vi "Check States.vi"(8 "error in (no error)":refnum<class "MultiErrors.lvclass">, 11 "Sequence Validation in":refnum<class "Sequence Validation.lvclass">) -> (0 "error out":refnum<class "MultiErrors.lvclass">, 3 "Sequence Validation out":refnum<class "Sequence Validation.lvclass">)   [LabVIEW 2020, in "VolatusSeq.lvlib" / "Sequence Validation.lvclass"]
uses:
  Sequence Validation.lvclass
  Sequence Validation.lvclass/Sequence Validation.ctl
  VolatusErrorUtilities/MultiErrors/MultiErrors.lvclass
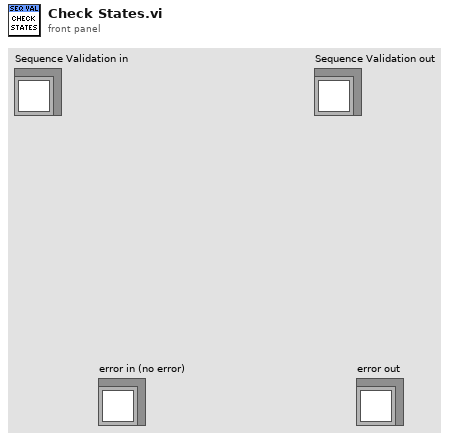
[diagram p1: front panel]
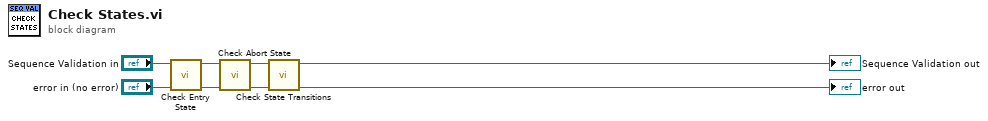
[diagram p0: block diagram]
diagram:
  n1 = call "Check Entry State.vi"("error in (no error)"="error in (no error)", "Sequence Validation in"="Sequence Validation in") -> ("error out"=w6:refnum<class "MultiErrors.lvclass">, "Sequence Validation out"=w5:refnum<class "Sequence Validation.lvclass">)  [unwired: 8 in]
  n2 = call "Check Abort State.vi"("error in (no error)"=w6, "Sequence Validation in"=w5) -> ("error out"=w3:refnum<class "MultiErrors.lvclass">, "Sequence Validation out"=w4:refnum<class "Sequence Validation.lvclass">)  [unwired: 8 in]
  n3 = call "Check State Transitions.vi"("error in (no error)"=w3, "Sequence Validation in"=w4) -> ("error out"=→"error out":refnum<class "MultiErrors.lvclass">, "Sequence Validation out"=→"Sequence Validation out":refnum<class "Sequence Validation.lvclass">)  [unwired: 8 in]
